vi "FlatToRichcif_manager_LoaderInfo.vi"(5 "OutputClusterType":T1, 11 "InputCluster":T3) -> (3 "OutputCluster":T1)   [LabVIEW 2021, in "CIF_PluginLoader_client.lvlib"]
uses:
  CIF_PluginLoader_client.lvlib
  cif_manager_LoaderInfo_Flat.ctl
  cif_manager_LoaderType.ctl
  cif_manager_LoaderInfo.ctl
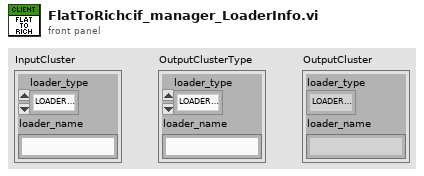
[diagram p1: front panel]
types:
  T1 = typedef "CIF_PluginLoader_client.lvlib/cif_manager_LoaderInfo.ctl" = cluster{"loader_type":T2, "loader_name":string}
  T2 = typedef "CIF_PluginLoader_client.lvlib/cif_manager_LoaderType.ctl" = enum32{"LOADERTYPE_UNKNOWN", "LOADERTYPE_LABVIEW"}
  T3 = typedef "CIF_PluginLoader_client.lvlib/cif_manager_LoaderInfo_Flat.ctl" = cluster{"loader_type":T2, "loader_name":string}
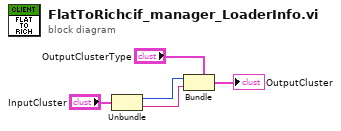
[diagram p0: block diagram]
diagram:
  n1 = Unbundle "Unbundle"("InputCluster") -> ("loader_type"=w2:T2, "loader_name"=w1:string)
  n2 = Bundle "Bundle"(cluster="OutputClusterType", "loader_type"=w2, "loader_name"=w1) -> (→"OutputCluster":T1)
